vi "PBKDF2 generator.vi"() -> ()   [LabVIEW 2020, in "wamplv.lvlib"]
uses:
  wamplv.lvlib
  Private/Utils/Utils.lvclass
panel:
  in  "Salt":string
  in  "Secret":string
  out "PBKDF2 result":string
  in  "Key Length":i32=32
  in  "Iterations":i32
  # "wamplv assumes PBKDF2 with SHA-256 hash, with the result represented as a lower case hex string"
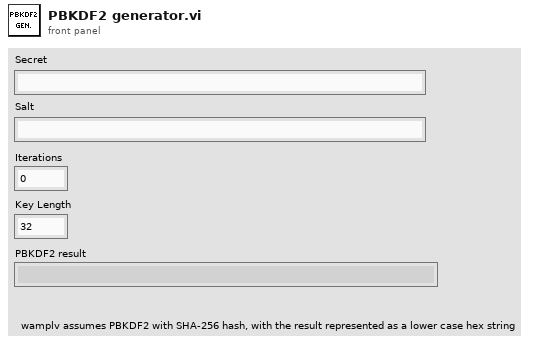
[diagram p1: front panel]
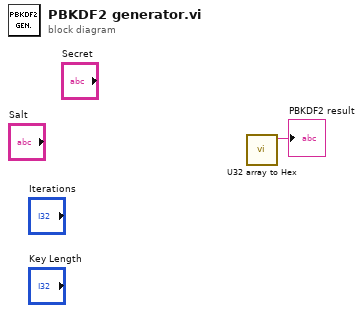
[diagram p0: block diagram]
diagram:
  n1 = call "U32 array to Hex.vi"() -> ("Hex string"=→"PBKDF2 result":string)  [unwired: 11 in]
